vi "chainCommands.vi"(9 "Command":string, 11 "StringIn":string) -> (3 "StringOut":string)   [LabVIEW 2012]
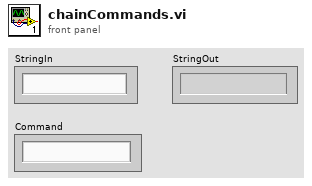
[diagram p1: front panel]
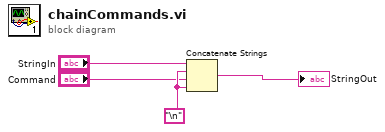
[diagram p0: block diagram]
diagram:
  w4 = "\n"
  n1 = Concatenate Strings("StringIn", w4, "Command", w4) -> (→"StringOut":string)
